vi "Fetch Measurement (Read) Hioky.vi"(8 "error in (no error)":errorcluster, 10 "Timeout (10000 ms)":u32=10000, 11 "VISA resource name":refnum<visa-resource-name>) -> (0 "error out":errorcluster, 1 "End of Data?":bool, 2 "Measurements":dbl[](array[numeric]), 3 "VISA resource name out":refnum<visa-resource-name>)   [LabVIEW 2017]
doc: "Fetches measurement from the instrument. This VI is to be used after \"READ?\" has been called. The VI will retrieve up to 10 data data points from the instrument's output buffer. This VI should be called repeatedly until End of Data? is True.\n\n<B>Note:</B>\n\nThis VI is called by <B>Fetch Measurement VI</B> in the following cases:\n(1) Model = 34401, Trigger Source = Immediate/External, and Math = Off/Output Buffer\n(2) Model = 34410/34411, Trigger Source = Immediate/External/Internal, and Math = On"
panel:
  out "return count":u32
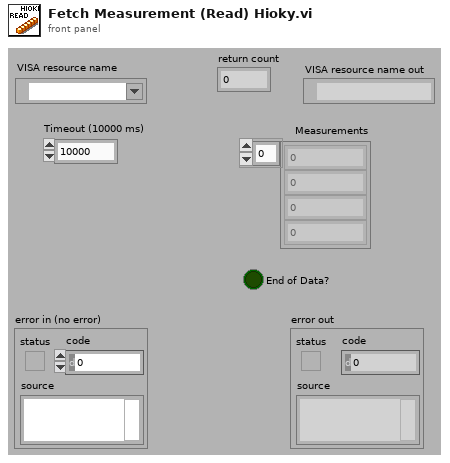
[diagram p1: front panel]
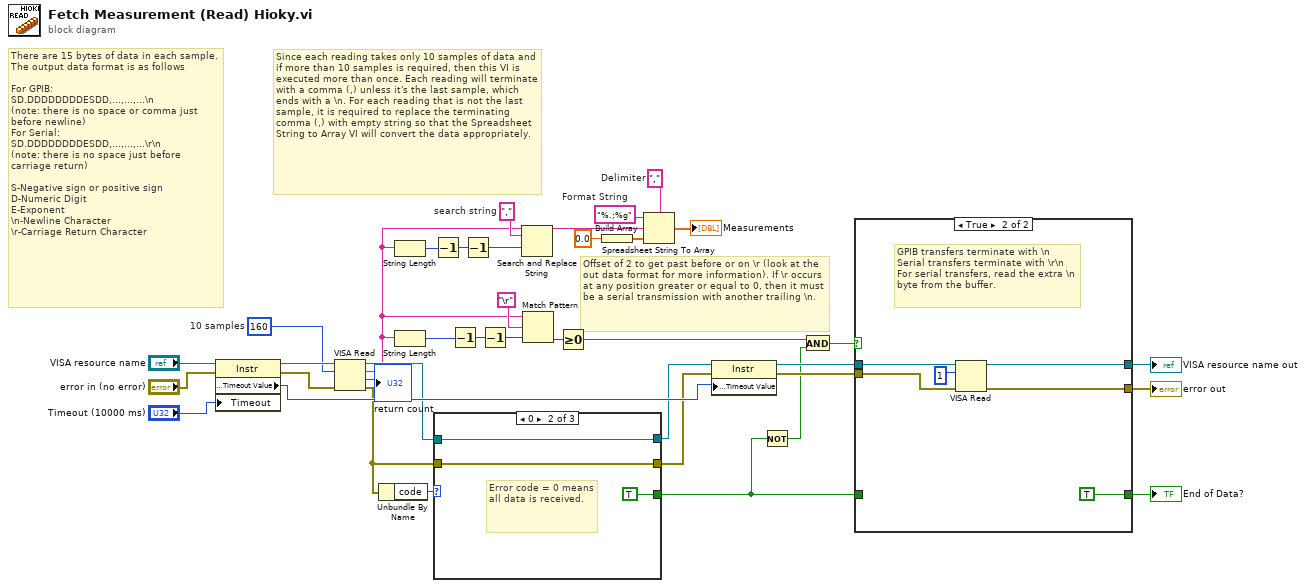
[diagram p0: block diagram]
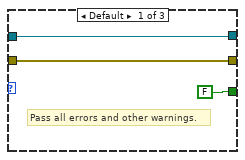
[diagram p2: hidden frame]
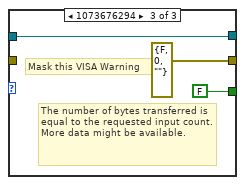
[diagram p3: hidden frame]
diagram:
  w27 = ","  # search string
  w37 = ","  # Delimiter
  w38 = "%.;%g"  # Format String
  w3 = u32 160  # 10 samples
  # "Offset of 2 to get past before or on \\r (look at the out data format for more information). If \\r occurs at any position greater or equal to 0, then it must be a serial transmission with another trailing \\n."
  # "Since each reading takes only 10 samples of data and if more than 10 samples is required, then this VI is executed more than once. Each reading will terminate with a comma (,) unless it's the last sample, which ends with a \\n. For each reading that is not the last sample, it is required to replace the terminating comma (,) with empty string so that the Spreadsheet String to Array VI will convert the data appropriately."
  # "There are 15 bytes of data in each sample. The output data format is as follows\n\nFor GPIB:\nSD.DDDDDDDDESDD,...,...,...\\n\n(note: there is no space or comma just before newline) \nFor Serial: \nSD.DDDDDDDDESDD,...,...,...\\r\\n\n(note: there is no space just before carriage return)\n\nS-Negative sign or positive sign\nD-Numeric Digit\nE-Exponent\n\\n-Newline Character\n\\r-Carriage Return Character"
  n1 = property on="Property Node" class="Instr"(reference="VISA resource name", error in="error in (no error)", "Timeout"="Timeout (10000 ms)") -> (reference out=w31:refnum<visa-resource-name>, error out=w30:errorcluster, "General Settings:Timeout Value"=w29:u32)
  n2 = VISA Read(VISA resource name=w31, byte count=w3, error in (no error)=w30) -> (VISA resource name out=w5:refnum<visa-resource-name>, read buffer=w2:string, return count=→"return count":u32, error out=w14:errorcluster)
  n3 = Unbundle By Name(w14) -> ("code"=w15:i32)
  n4 = String Length(string=w2) -> (length=w24:i32)
  n5 = String Length(string=w2) -> (length=w19:i32)
  n6 = Decrement(x=w24) -> (x-1=w25:i32)
  n7 = case shown="0" w15 {
    tunnel: w14 -> [w41 w42 _]
    tunnel: [w41 w42 errorcluster {"status"=FALSE, "code"=0, "source"=""} ("error out")] -> w13
    tunnel: [FALSE TRUE FALSE] -> w9
    tunnel: w5 -> [w39 w43 w45]
    tunnel: [w39 w43 w45] -> w4
    frame Default {
      # "Pass all errors and other warnings."
    }
    frame 0 {
      # "Error code = 0 means all data is received."
    }
    frame 1073676294 {
      # "Mask this VISA Warning"
      # "The number of bytes transferred is equal to the requested input count. More data might be available."
    }
  }
  n8 = Decrement(x=w19) -> (x-1=w20:i32)
  n9 = Decrement(x=w25) -> (x-1=w23:i32)
  n10 = Decrement(x=w20) -> (x-1=w18:i32)
  n11 = Search and Replace String(input string=w2, search string=w27, offset=w23) -> (result string=w26:string)  [unwired: 5 in, 3 out]
  n12 = Match Pattern(string=w2, regular expression="\r" ("Carriage Return Constant"), offset (0)=w18) -> (offset past match=w21:i32)  [unwired: 3 out]
  n13 = Greater Or Equal To 0?(x=w21) -> (x >= 0?=w11:bool)
  n14 = Build Array(0.0) -> (w35:dbl[])
  n15 = Spreadsheet String To Array(delimiter (Tab)=w37, format string=w38, spreadsheet string=w26, array type (2D Dbl)=w35) -> (array=→"Measurements":dbl[])
  n16 = property on="Property Node" class="Instr"(reference=w4, error in=w13, "General Settings:Timeout Value"=w29) -> (reference out=w17:refnum<visa-resource-name>, error out=w16:errorcluster)
  n17 = Not(x=w9) -> (.not. x?=w10:bool)
  n18 = And(x=w11, y=w10) -> (x .and. y?=w12:bool)
  n19 = case shown="True" w12 {
    tunnel: w17 -> [w50 w56]
    tunnel: w16 -> [w49 w55]
    tunnel: [w50 w53] -> w6
    tunnel: [w49 w51] -> w7
    tunnel: w9 -> [w48 _]
    tunnel: [w48 TRUE] -> w8
    frame False {
      # "For GPIB transfers, error condition, or incomplete serial operations, pass VISA session, error cluster and previously determined End of Data Boolean."
    }
    frame True {
      # "GPIB transfers terminate with \\n\nSerial transfers terminate with \\r\\n\nFor serial transfers, read the extra \\n byte from the buffer."
      n20 = VISA Read(VISA resource name=w56, byte count=u32 1, error in (no error)=w55) -> (VISA resource name out=w53:refnum<visa-resource-name>, error out=w51:errorcluster)  [unwired: 2 out]
    }
  }
  "VISA resource name out" <- w6
  "error out" <- w7
  "End of Data?" <- w8
